vi "Problem1.12-NoSubVI.vi"() -> ()   [LabVIEW 2019]
panel:
  out "g":dbl
  out "s":dbl
  out "Uniform Deviate  2":dbl
  out "Uniform Deviate 1":dbl
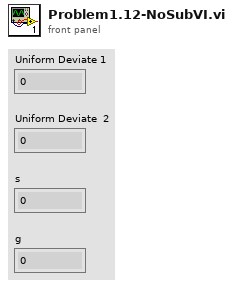
[diagram p1: front panel]
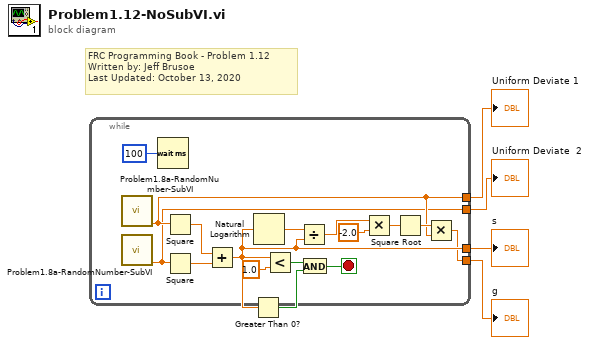
[diagram p0: block diagram]
diagram:
  # "FRC Programming Book - Problem 1.12\nWritten by: Jeff Brusoe\nLast Updated: October 13, 2020"
  n1 = while {
    tunnel: [w8] -> w4
    tunnel: [w7] -> w3
    tunnel: [w6] -> w2
    tunnel: [w5] -> w1
    stop <- w20 stop-if-true
    n2 = call "Problem1.8a-RandomNumber-SubVI.vi"() -> ("Uniform Deviate"=w8:dbl)  [unwired: 10 in, 1 out]
    n3 = call "Problem1.8a-RandomNumber-SubVI.vi"() -> ("Uniform Deviate"=w7:dbl)  [unwired: 10 in, 1 out]
    n4 = Wait (ms)(milliseconds to wait=u32 100) -> ()  [unwired: 1 out]
    n5 = Square(x=w8) -> (x^2=w16:dbl)
    n6 = Square(x=w7) -> (x^2=w15:dbl)
    n7 = Add(x=w16, y=w15) -> (x+y=w6:dbl)
    n8 = Greater Than 0?(x=w6) -> (x > 0?=w19:bool)
    n9 = Natural Logarithm(1:w6) -> (0:w13:dbl)
    n10 = Less?(x=w6, y=1.0) -> (x < y?=w18:bool)
    n11 = Divide(x=w13, y=w6) -> (x/y=w12:dbl)
    n12 = And(x=w18, y=w19) -> (x .and. y?=w20:bool)
    n13 = Multiply(x=w12, y=-2.0) -> (x*y=w10:dbl)
    n14 = Square Root(x=w10) -> (sqrt(x)=w9:dbl)
    n15 = Multiply(x=w9, y=w8) -> (x*y=w5:dbl)
  }
  "Uniform Deviate 1" <- w4
  "Uniform Deviate  2" <- w3
  "s" <- w2
  "g" <- w1
